vi "main_user.vi"() -> ()   [LabVIEW 2017]
uses:
  <vilib>/ErrorRing/Error Ring.xnode
  <vilib>/measure/NI_MABase.lvlib
panel:
  in  "Offset [V]":dbl(slide) min=-5.0 max=5.0 scale=-5.0..5.0 scale format="%.1g"
  out "Período":dbl
  in  "Frequência":dbl
  in  "Ciclos":dbl
  in  "Stop Button":bool
  in  "Amplitude [V]":dbl(slide) min=0.0 max=10.0 scale=0.0..10.0 scale format="%.2g"
  in  "Tipo de forma de onda":T1(ring)
  in  "Play Button":bool
  out "Waveform Chart":waveform(dbl)(graph) caption="Sinal gerado"
  # "Gerador de Funções"
  # "Selecione a forma de    onda, frequência e    amplitude e clique em 'Play' para visualizar a forma de onda. \n   Clique em 'Stop' para sair."
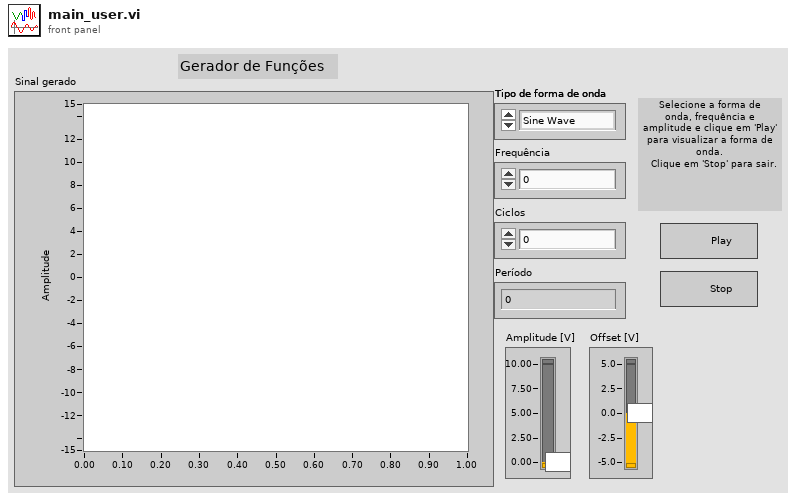
[diagram p1: front panel]
types:
  T1 = enum16{"Sine Wave", "Triangle Wave", "Square Wave", "Sawtooth Wave"}
  T2 = enum16{"Wait for event", "Stop", "Clean Graph", "Waveform", "Initialize"}
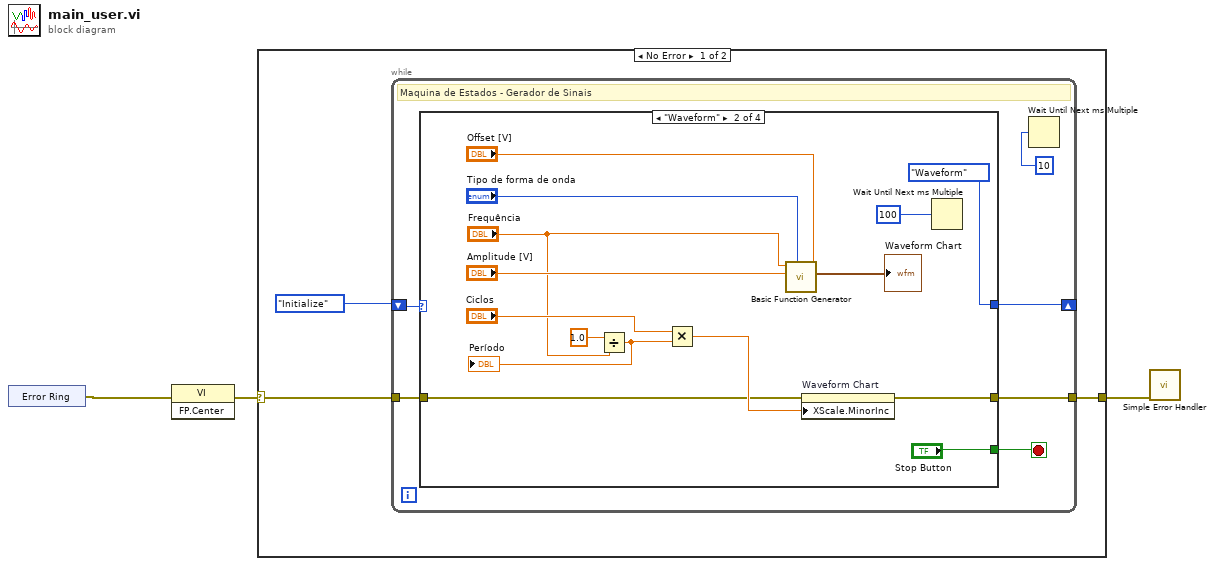
[diagram p0: block diagram]
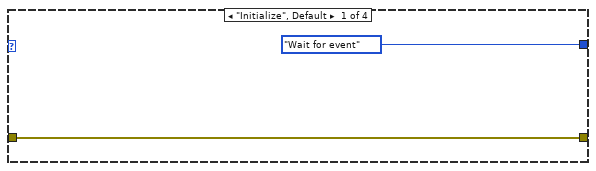
[diagram p2: hidden frame]
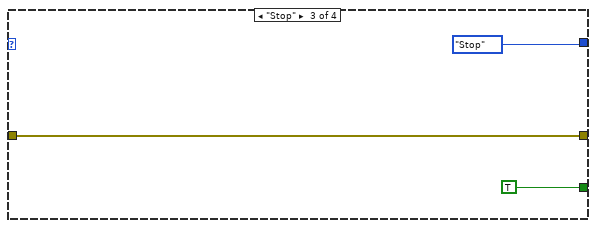
[diagram p3: hidden frame]
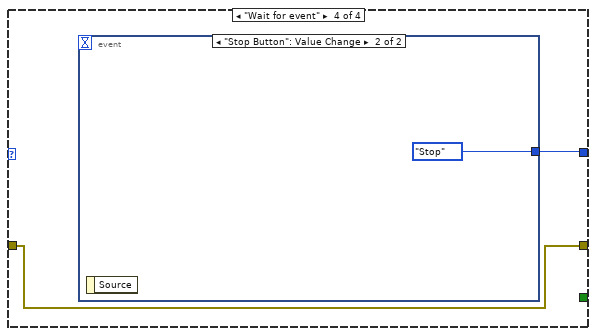
[diagram p4: hidden frame]
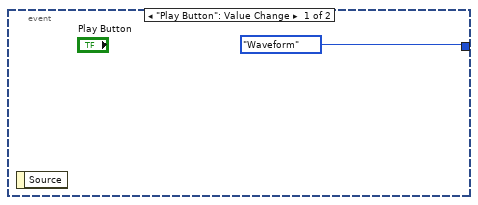
[diagram p5: hidden frame]
diagram:
  n1 = xnode "Error Ring"() -> ("error out"=w2:errorcluster)
  n2 = invoke class="VI" method="FP.Center"(error in=w2) -> (error out=w1:errorcluster)  [unwired: 2 in, 2 out]
  n3 = case shown="No Error" w1 {
    selector: w1 -> [w5 w36]
    tunnel: [w4 w36] -> w3
    frame No Error {
      n4 = while {
        shift-right: [w11] -> _
        shift-left: T2."Initialize" -> [w12]
        tunnel: [w8] -> w4
        tunnel: w5 -> [w7]
        stop <- w10 stop-if-true
        # "Maquina de Estados - Gerador de Sinais"
        n5 = case shown="\"Waveform\"" w12 {
          tunnel: [T2."Wait for event" T2."Waveform" T2."Stop" w33] -> w11
          tunnel: [_ "Stop Button" TRUE _] -> w10
          tunnel: [w13 w17 w29 w32] -> w8
          tunnel: w7 -> [w13 w16 w29 w32]
          frame "Initialize", Default {
          }
          frame "Waveform" {
            n6 = Divide(x=1.0, y="Frequência") -> (x/y=w19:dbl)
            "Período" <- w19
            n7 = Multiply(x="Ciclos", y=w19) -> (x*y=w18:dbl)
            n8 = call <vilib>:"Basic Function Generator.vi"("offset"="Offset [V]", "signal type"="Tipo de forma de onda", "amplitude"="Amplitude [V]", "frequency"="Frequência") -> ("signal out"=→"Waveform Chart":waveform(dbl))  [unwired: 5 in, 2 out]
            n9 = property on="Waveform Chart" class="WFChart (strict)"(error in=w16, "XScale.MinorInc"=w18) -> (error out=w17:errorcluster)  [unwired: 1 in, 1 out]
            n10 = Wait Until Next ms Multiple(millisecond multiple=u32 100) -> ()  [unwired: 1 out]
          }
          frame "Stop" {
          }
          frame "Wait for event" {
            n11 = event shown="[1] \"Stop Button\": Value Change" {
              selector: _ -> [_ _]
              dyn-events: _ -> [_ _]
              timeout: _ -> [_ _]
              tunnel: [T2."Waveform" T2."Stop"] -> w33
              event "Play Button": Value Change {
                n12 = event-data() -> ()  [unwired: 1 in, 1 out]
              }
              event "Stop Button": Value Change {
                n13 = event-data() -> ()  [unwired: 1 in, 1 out]
              }
            }
          }
        }
        n14 = Wait Until Next ms Multiple(millisecond multiple=u32 10) -> ()  [unwired: 1 out]
      }
    }
    frame Error {
    }
  }
  n15 = call <vilib>:"Simple Error Handler.vi"("error in (no error)"=w3) -> ()  [unwired: 4 in, 5 out]
